vi "Multilabel_Classification.vi"(8 "error in (no error)":errorcluster caption="entrée d'erreur (pas d'erreur)", 11 "make_multilabel_classification":T2={"n_samples"=100, "n_features"=20, "n_classes"=5, "n_labels"=2, "length"=50, "allow_unlabeled"=TRUE, "sparse"=FALSE, "return_indicator"="dense", "random_state"=-1, "Returns"="X"} {"random_state" min=-1; "length" min=1; "n_classes" min=1; "n_features" min=1; "n_samples" min=1}) -> (0 "error out":errorcluster, 3 "Data":T1)   [LabVIEW 2020]
doc: "Generate a random multilabel classification problem.\n\nFor each sample, the generative process is :\n\n- pick the number of labels: n ~ Poisson(n_labels)\n- n times, choose a class c: c ~ Multinomial(theta)\n- pick the document length: k ~ Poisson(length)\n- k times, choose a word: w ~ Multinomial(theta_c)\n\nIn the above process, rejection sampling is used to make sure that n is never zero or more than n_classes, and that the document length is never zero. Likewise, we reject classes which have already been chosen.\n\n\n\nParameters :\n\n- n_samples : int, optional (default=100)\nThe number of samples.\n\n- n_features : int, optional (default=20)\nThe total number of features.\n\n- n_classes : int, optional (default=5)\nThe number of classes of the classification problem.\n\n- n_labels : int, optional (default=2)\nThe average number of labels per instance. More precisely, the number of labels per sample is drawn from a Poisson distribution with n_labels as its expected value, but samples are bounded (using rejection sampling) by n_classes, and must be nonzero if allow_unlabeled is False.\n\n- length : int, optional (default=50)\nThe sum of the features (number of words if documents) is drawn from a Poisson distribution with this expected value.\n\n- allow_unlabeled : bool, optional (default=True)\nIf True, some instances might not belong to any class.\n\n- sparse : bool, optional (default=False)\nIf True, return a sparse feature matrix\n\n- return_indicator : ‘dense’ (default) | ‘sparse’ | False\nIf dense return Y in the dense binary indicator format. If 'sparse' return Y in the sparse binary indicator format. False returns a list of lists of labels.\n\n- random_state : int, RandomState instance, default=None=-1\nDetermines random number generation for dataset creation. Pass an int for reproducible output across multiple function calls. See Glossary.\n\nReturns : \n\n- X : array of shape [n_samples, n_features]\nThe generated samples.\n\n- Y : array or sparse CSR matrix of shape [n_samples, n_classes]\nThe label sets.\n\n- p_c : array, shape [n_classes]\nThe probability of each class being drawn. Only returned if return_distributions=True.\n\n- p_w_c : array, shape [n_features, n_classes]\nThe probability of each feature being drawn given each class. Only returned if return_distributions=True."
uses:
  Multilabel_Classification.lvclass
panel:
  out "Multilabel_Classification.lvclass":refnum<class "Multilabel_Classification.lvclass">
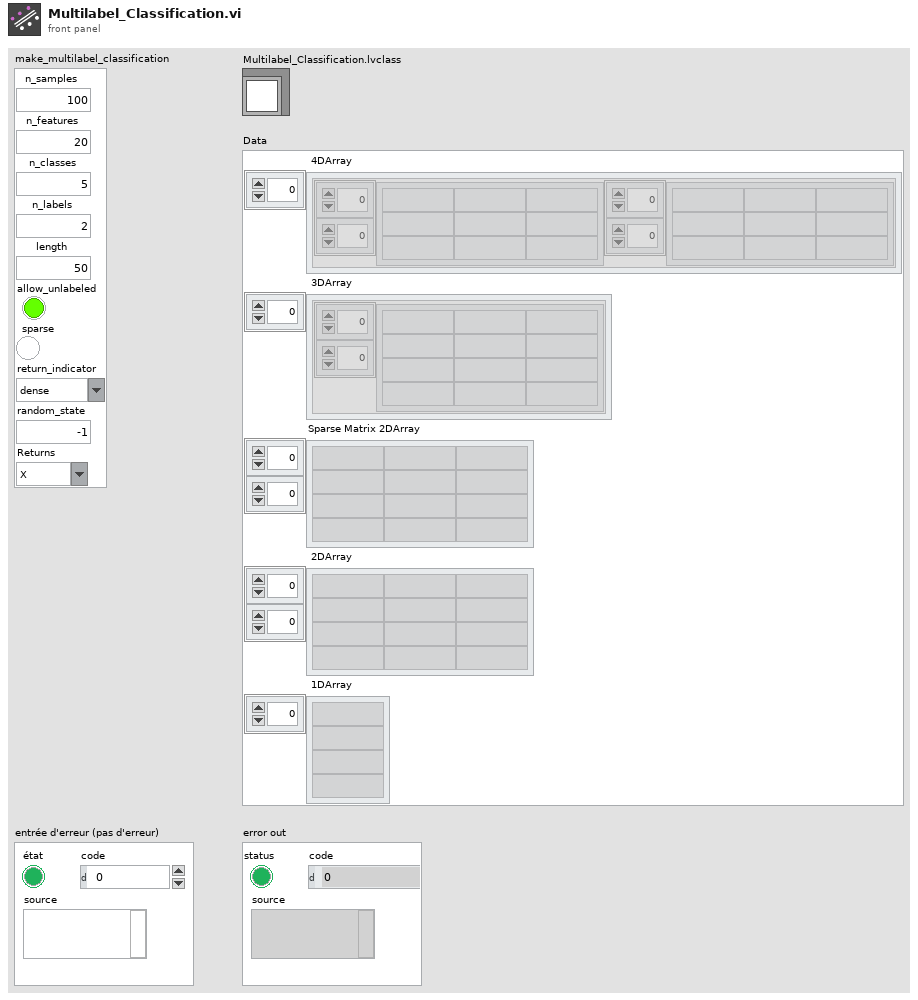
[diagram p1: front panel]
types:
  T1 = cluster{" 4DArray":cluster{"1":string[][], "2":string[][]}[], " 3DArray":cluster{"Tableau":string[][]}[], "Sparse Matrix 2DArray":string[][], " 2DArray":string[][], " 1DArray":string[]}
  T2 = cluster{"n_samples":u32, "n_features":u32, "n_classes":u32, "n_labels":u32, "length":u32, "allow_unlabeled":bool, "sparse":bool, "return_indicator":string, "random_state":i32, "Returns":string}
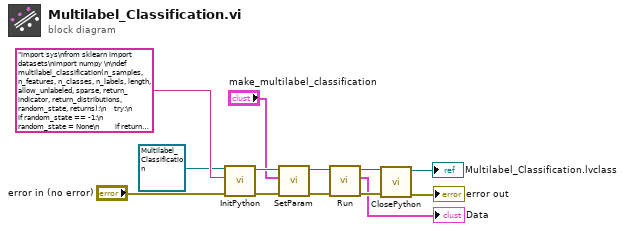
[diagram p0: block diagram]
diagram:
  n1 = call-dynamic "InitPython.vi"("error in (no error)"="error in (no error)", "Python Instruction"="import sys\nfrom sklearn import datasets\nimport numpy \n\ndef multilabel_classification(n_samples, n_features, n_classes, n_labels, length, allow_unlabeled, sparse, return_indicator, return_distributions, random_state, returns):\n    try:\n        if random_state == -1:\n            random_state = None\n        if return_indicator == 'False':\n            return_indicator = False\n        X, y, p_c, p_w_c = datasets.make_multilabel_classification(n_samples, n_features, n_classes, n_labels, length, allow_unlabeled, sparse, return_indicator, return_distributions, random_state)\n        dtype = type(y) \n        if returns == 'X':\n            dataX = X.tolist()\n            return str(dataX)\n        elif returns == 'Y':\n            if dtype == numpy.ndarray:\n                datay = y.tolist()\n                return str(datay)\n            else:\n                Mat = y.tocoo()\n                return str(list(zip(Mat.row, Mat.col, Mat.data)))\n        elif returns == 'p_c':\n            data_p_c = p_c.tolist()\n            return str(data_p_c)\n        else:\n            data_p_w_c = p_w_c.tolist()\n            return str(data_p_w_c)\n    except:\n        erreur = sys.exc_info()\n        typerr = u\"%s\" % (erreur[0])\n        typerr = typerr[typerr.find(\"'\")+1:typerr.rfind(\"'\")]\n        msgerr = u\"%s\" % (erreur[1])\n        message = str('/!\\\\ {0} : {1}'. format(typerr,msgerr))\n        return message", "Scikit-learn en entrée"=refnum<class "Multilabel_Classification.lvclass"> refnum ("Multilabel_Classification.lvclass")) -> ("error out"=w9:errorcluster, "Scikit-learn en sortie"=w10:refnum<class "Multilabel_Classification.lvclass">)  [unwired: 7 in]
  n2 = call-dynamic "SetParam.vi"("error in (no error)"=w9, "make_multilabel_classification"="make_multilabel_classification", "Multilabel_Classification.lvclass"=w10) -> ("error out"=w6:errorcluster, "Multilabel_Classification.lvclass"=w7:refnum<class "Multilabel_Classification.lvclass">)  [unwired: 7 in]
  n3 = call-dynamic "Run.vi"("error in (no error)"=w6, "Multilabel_Classification.lvclass"=w7) -> ("error out"=w4:errorcluster, "Data"=→"Data":T1, "Multilabel_Classification.lvclass"=w5:refnum<class "Multilabel_Classification.lvclass">)  [unwired: 7 in]
  n4 = call-dynamic "ClosePython.vi"("error in (no error)"=w4, "Scikit-learn en entrée"=w5) -> ("error out"=→"error out":errorcluster, "Scikit-learn en sortie"=→"Multilabel_Classification.lvclass":refnum<class "Multilabel_Classification.lvclass">)  [unwired: 8 in]
